vi "TC_to_DSC.vi"(8 "error in (no error)":errorcluster, 11 "TC Cluster":T1) -> (0 "error out":errorcluster)   [LabVIEW 2016]
uses:
  Typedefs/TC-cluster.ctl
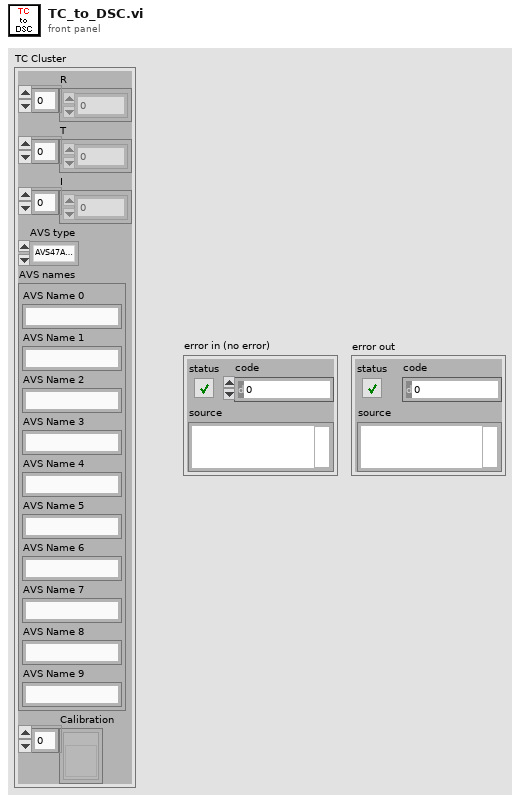
[diagram p1: front panel]
types:
  T1 = typedef "TC-cluster.ctl" = cluster{"R":dbl[], "T":dbl[], "I":dbl[], "AVS type":enum16{"AVS47A (GPIB interface)", "AVS47B (RS232 interface)", "AVS48", "AVS Emulation", "Impedance Bridge", "Disabled"}, "AVS names":cluster{"AVS Name 0":string, "AVS Name 1":string, "AVS Name 2":string, "AVS Name 3":string, "AVS Name 4":string, "AVS Name 5":string, "AVS Name 6":string, "AVS Name 7":string, "AVS Name 8":string, "AVS Name 9":string}, "Calibration":refnum<vi>[]}
  T2 = enum16{"AVS47A (GPIB interface)", "AVS47B (RS232 interface)", "AVS48", "AVS Emulation", "Impedance Bridge", "Disabled"}
  T3 = cluster{"AVS Name 0":string, "AVS Name 1":string, "AVS Name 2":string, "AVS Name 3":string, "AVS Name 4":string, "AVS Name 5":string, "AVS Name 6":string, "AVS Name 7":string, "AVS Name 8":string, "AVS Name 9":string}
  T4 = enum16{"CF", "CF_Z_Bridge", "MNK", "MNK_Z_Bridge"}
  T5 = cluster{"[0]":string, "[1]":string, "[2]":string, "[3]":string, "[4]":string, "[5]":string, "[6]":string, "[7]":string, "[8]":string, "[9]":string}
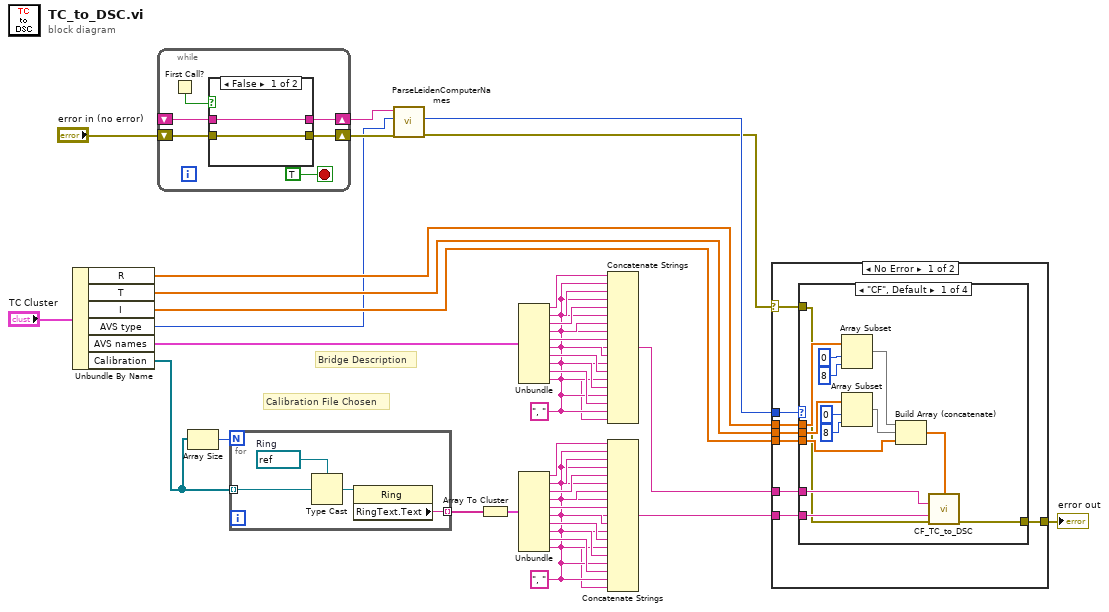
[diagram p0: block diagram]
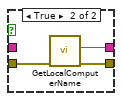
[diagram p2: hidden frame]
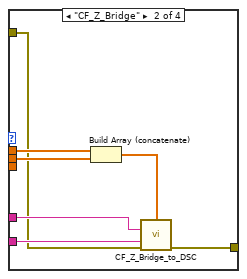
[diagram p3: hidden frame]
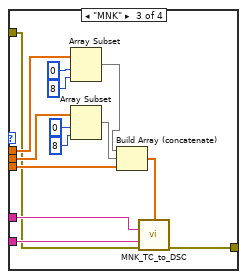
[diagram p4: hidden frame]
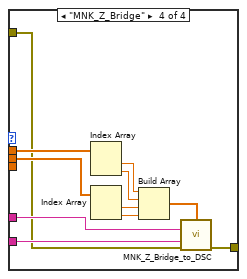
[diagram p5: hidden frame]
diagram:
  w17 = ", " ("string")
  w31 = ", " ("string")
  # "Bridge Description"
  # "Calibration File Chosen"
  n1 = Unbundle By Name("TC Cluster") -> ("R"=w6:dbl[], "T"=w5:dbl[], "I"=w4:dbl[], "AVS type"=w3:T2, "AVS names"=w2:T3, "Calibration"=w1:refnum<vi>[])
  n2 = while {
    shift-right: [w45] -> w10
    shift-left: "error in (no error)" -> [w42]
    shift-right: [w46] -> w12
    shift-left: _ -> [w41]
    stop <- TRUE stop-if-true
    n3 = First Call?() -> (First Call?: T/F=w44:bool)
    n4 = case shown="False" w44 {
      tunnel: [w48 w51] -> w46
      tunnel: [w47 w50] -> w45
      tunnel: w42 -> [w47 w49]
      tunnel: w41 -> [w48 _]
      frame False {
      }
      frame True {
        n5 = call "GetLocalComputerName.vi"("error in (no error)"=w49) -> ("error out"=w50:errorcluster, "Name"=w51:string)  [unwired: 8 in, 1 out]
      }
    }
  }
  n6 = Array Size(array=w1) -> (size(s)=w28:i32)
  n7 = for {
    N: w28 -> [_]
    tunnel: w1 -> [w55] mode=indexing
    tunnel: [w52] -> w27 mode=indexing
    w54 = refnum<vi> refnum  # Ring
    n8 = Type Cast(type=w54, x=w55) -> (*(type *) &x=w53:refnum<vi>)
    n9 = property class="Ring"(reference=w53) -> ("RingText.Text"=w52:string)  [unwired: 1 in, 2 out]
  }
  n10 = call "ParseLeidenComputerNames.vi"("error in (no error)"=w10, "AVS type"=w3, "computer name"=w12) -> ("error out"=w11:errorcluster, "AVS Type"=w13:T4)  [unwired: 6 in, 1 out]
  n11 = Array To Cluster(array=w27) -> (cluster=w15:T5)
  n12 = Unbundle(w2) -> ("AVS Name 0"=w40:string, "AVS Name 1"=w39:string, "AVS Name 2"=w38:string, "AVS Name 3"=w37:string, "AVS Name 4"=w36:string, "AVS Name 5"=w35:string, "AVS Name 6"=w34:string, "AVS Name 7"=w33:string, "AVS Name 8"=w32:string, "AVS Name 9"=w30:string)
  n13 = Unbundle(w15) -> ("[0]"=w26:string, "[1]"=w25:string, "[2]"=w24:string, "[3]"=w23:string, "[4]"=w22:string, "[5]"=w21:string, "[6]"=w20:string, "[7]"=w19:string, "[8]"=w18:string, "[9]"=w16:string)
  n14 = Concatenate Strings(w40, w31, w39, w31, w38, w31, w37, w31, w36, w31, w35, w31, w34, w31, w33, w31, w32, w31, w30) -> (w29:string)
  n15 = Concatenate Strings(w26, w17, w25, w17, w24, w17, w23, w17, w22, w17, w21, w17, w20, w17, w19, w17, w18, w17, w16) -> (w14:string)
  n16 = case shown="No Error" w11 {
    selector: w11 -> [w57 w110]
    tunnel: w29 -> [w63 _]
    tunnel: w14 -> [w62 _]
    tunnel: w13 -> [w61 _]
    tunnel: w6 -> [w60 _]
    tunnel: w5 -> [w59 _]
    tunnel: w4 -> [w58 _]
    tunnel: [w56 w110] -> w8
    frame No Error {
      n17 = case shown="\"CF\", Default" w61 {
        tunnel: w60 -> [w66 w84 w90 w108]
        tunnel: w59 -> [w69 w83 w89 w109]
        tunnel: w58 -> [w70 _ w98 _]
        tunnel: w63 -> [w77 w82 w96 w102]
        tunnel: w62 -> [w76 w81 w97 w101]
        tunnel: w57 -> [w64 w79 w86 w100]
        tunnel: [w65 w78 w85 w99] -> w56
        frame "CF", Default {
          n18 = Array Subset(array=w66, index=0, length=8) -> (w68:dbl[])
          n19 = Array Subset(array=w69, index=0, length=8) -> (w67:dbl[])
          n20 = Build Array (concatenate)(w68, w67, w70) -> (w75:dbl[])
          n21 = call "CF_TC_to_DSC.vi"("dbl"=w75, "String In"=w77, "String In 2"=w76, "error in (no error)"=w64) -> ("error out"=w65:errorcluster)  [unwired: 11 in]
        }
        frame "CF_Z_Bridge" {
          n22 = Build Array (concatenate)(w84, w83) -> (w80:dbl[])
          n23 = call "CF_Z_Bridge_to_DSC.vi"("dbl"=w80, "String In"=w82, "String In 2"=w81, "error in (no error)"=w79) -> ("error out"=w78:errorcluster)  [unwired: 11 in]
        }
        frame "MNK" {
          n24 = Array Subset(array=w90, index=0, length=8) -> (w87:dbl[])
          n25 = Array Subset(array=w89, index=0, length=8) -> (w88:dbl[])
          n26 = Build Array (concatenate)(w87, w88, w98) -> (w95:dbl[])
          n27 = call "MNK_TC_to_DSC.vi"("dbl"=w95, "String In"=w96, "String In 2"=w97, "error in (no error)"=w86) -> ("error out"=w85:errorcluster)  [unwired: 11 in]
        }
        frame "MNK_Z_Bridge" {
          n28 = Index Array(array=w108) -> (element #1=w107:dbl, element #2=w106:dbl)  [unwired: 2 in]
          n29 = Index Array(array=w109) -> (element #1=w105:dbl, element #2=w104:dbl)  [unwired: 2 in]
          n30 = Build Array(w107, w106, w105, w104) -> (w103:dbl[])
          n31 = call "MNK_Z_Bridge_to_DSC.vi"("dbl"=w103, "String In"=w102, "String In 2"=w101, "error in (no error)"=w100) -> ("error out"=w99:errorcluster)  [unwired: 11 in]
        }
      }
    }
    frame Error {
    }
  }
  "error out" <- w8
